vi "IsItemDecendant.vi"(8 "error in (no error)":errorcluster, 9 "Item to compare":refnum<class "ILabVIEWItem.lvclass">, 10 "Parent check?":bool, 11 "CLabVIEWItem in":refnum<class "CLabVIEWItem.lvclass">) -> (0 "error out":errorcluster, 2 "Is a decendant?":bool, 3 "CLabVIEWItem out":refnum<class "CLabVIEWItem.lvclass">)   [LabVIEW 2020, in "LabVIEWItem.lvlib" / "CLabVIEWItem.lvclass"]
uses:
  CLabVIEWItem.lvclass
  obj/Addons/LabVIEWObjectInterfaces.lvlibp/LabVIEWObjectInterfaces/ILabVIEWItem/ILabVIEWItem.lvclass
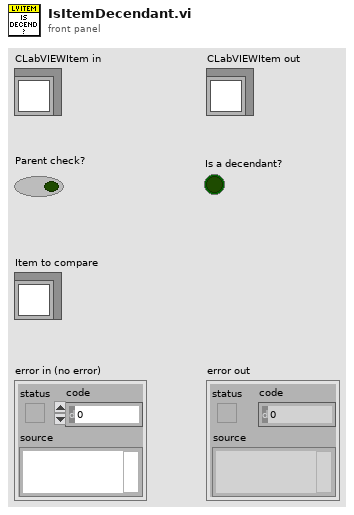
[diagram p1: front panel]
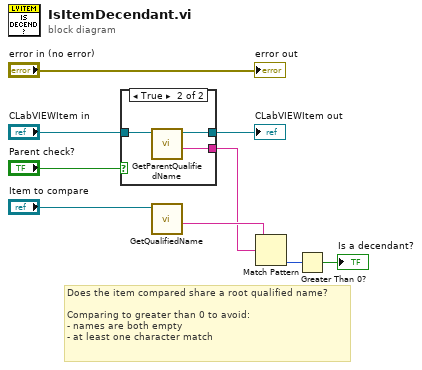
[diagram p0: block diagram]
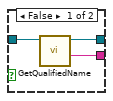
[diagram p2: hidden frame]
diagram:
  # "Does the item compared share a root qualified name?\n\nComparing to greater than 0 to avoid:\n- names are both empty\n- at least one character match"
  n1 = case shown="True" "Parent check?" {
    tunnel: "CLabVIEWItem in" -> [w12 w15]
    tunnel: [w11 w14] -> w7
    tunnel: [w10 w13] -> w3
    frame False {
      n2 = call-dynamic "GetQualifiedName.vi"("CLabVIEWItem in"=w12) -> ("Qualified name"=w10:string, "CLabVIEWItem out"=w11:refnum<class "CLabVIEWItem.lvclass">)  [unwired: 8 in, 1 out]
    }
    frame True {
      n3 = call-dynamic "GetParentQualifiedName.vi"("CLabVIEWItem in"=w15) -> ("Name"=w13:string, "CLabVIEWItem out"=w14:refnum<class "CLabVIEWItem.lvclass">)  [unwired: 8 in, 1 out]
    }
  }
  "CLabVIEWItem out" <- w7
  n4 = call-dynamic "GetQualifiedName.vi"("ILabVIEWItem in"="Item to compare") -> ("Qualified name"=w4:string)  [unwired: 8 in, 2 out]
  n5 = Match Pattern(string=w4, regular expression=w3) -> (offset past match=w9:i32)  [unwired: 1 in, 3 out]
  n6 = Greater Than 0?(x=w9) -> (x > 0?=→"Is a decendant?":bool)
  "error out" <- "error in (no error)"
